vi "Rawdata_Analyzer.vi"() -> ()   [LabVIEW 2020]
uses:
  ctl/Image_RAW_Bayer_Pattern.ctl
  ctl/Image_Configuration.ctl
  <vilib>/vision/Image Controls.llb/IMAQ Image.ctl
  <vilib>/Analysis/NI_AALBase.lvlib
panel:
  in  "stop":bool
  out "Current Color Histogram":cluster{"R":u8, "G":u8, "B":u8}
  out "Current Timestamp":u64
  out "Current Image":T1(plugin-control)
  out "Progress":dbl(slide) scale=0.0..100.0
  out "Frame Color Histogram":cluster{"R":u8, "G":u8, "B":u8}[](array[cluster])
  in  "Image Configuration":T2={"Width"=3840, "Height"=2160}
  in  "Bayer Pattern":T3=enum."RGGB (GRBG)"
  in  "Analyze Color?":bool
  in  "Analyze Timestamp?":bool=TRUE
  out "error out":errorcluster
  out "Frame Timestamp (ns)":u64[](array[numeric])
  out "Bytes per Frame":u32
  out "Total Frame Num":i64
  in  "RAWdata File Path":path
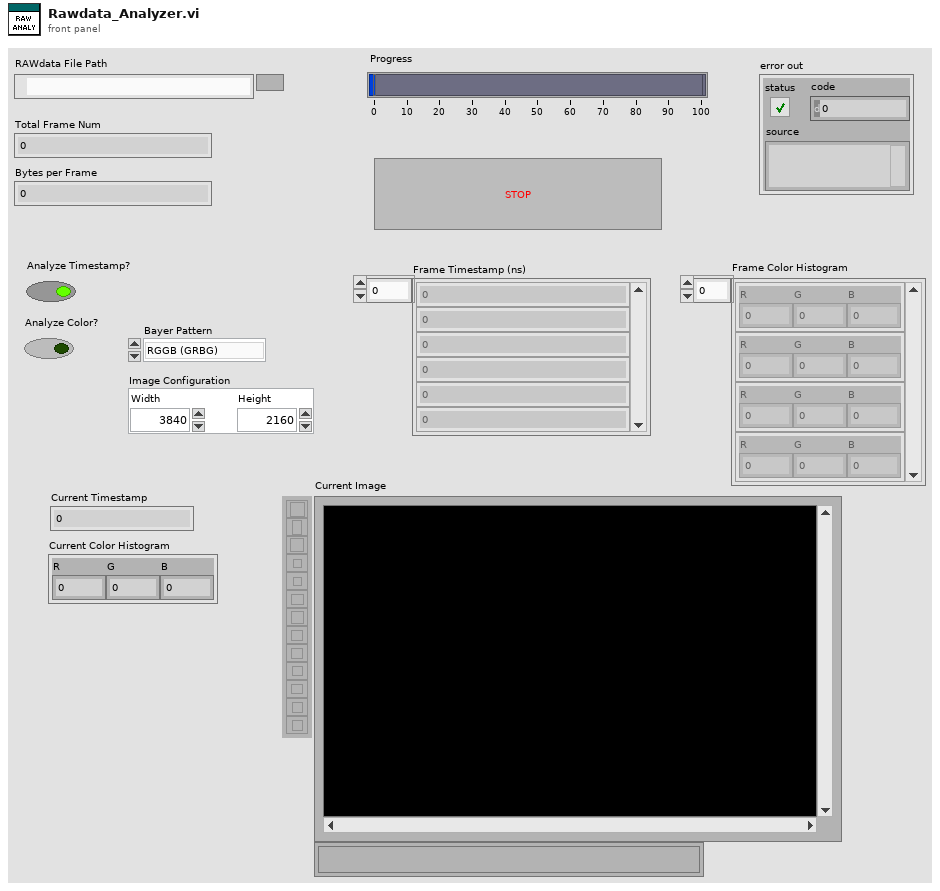
[diagram p1: front panel]
types:
  T1 = typedef "IMAQ Image.ctl" = refnum<image>
  T2 = typedef "Image_Configuration.ctl" = cluster{"Width":i32, "Height":i32}
  T3 = typedef "Image_RAW_Bayer_Pattern.ctl" = enum16{"GBRG (BGGR)", "GRBG (RGGB)", "BGGR (GBRG)", "RGGB (GRBG)", "CRBC (RCCB)"}
  T4 = typedef "Image_Data_Config.ctl" = cluster{"Lines of Image Data":u16, "Bytes per Even Line":u16, "Bytes per Odd Line":u16, "Image Data Type":u8, "Total Image Data Block Size":u32, "Image Data Block Offset":u32}
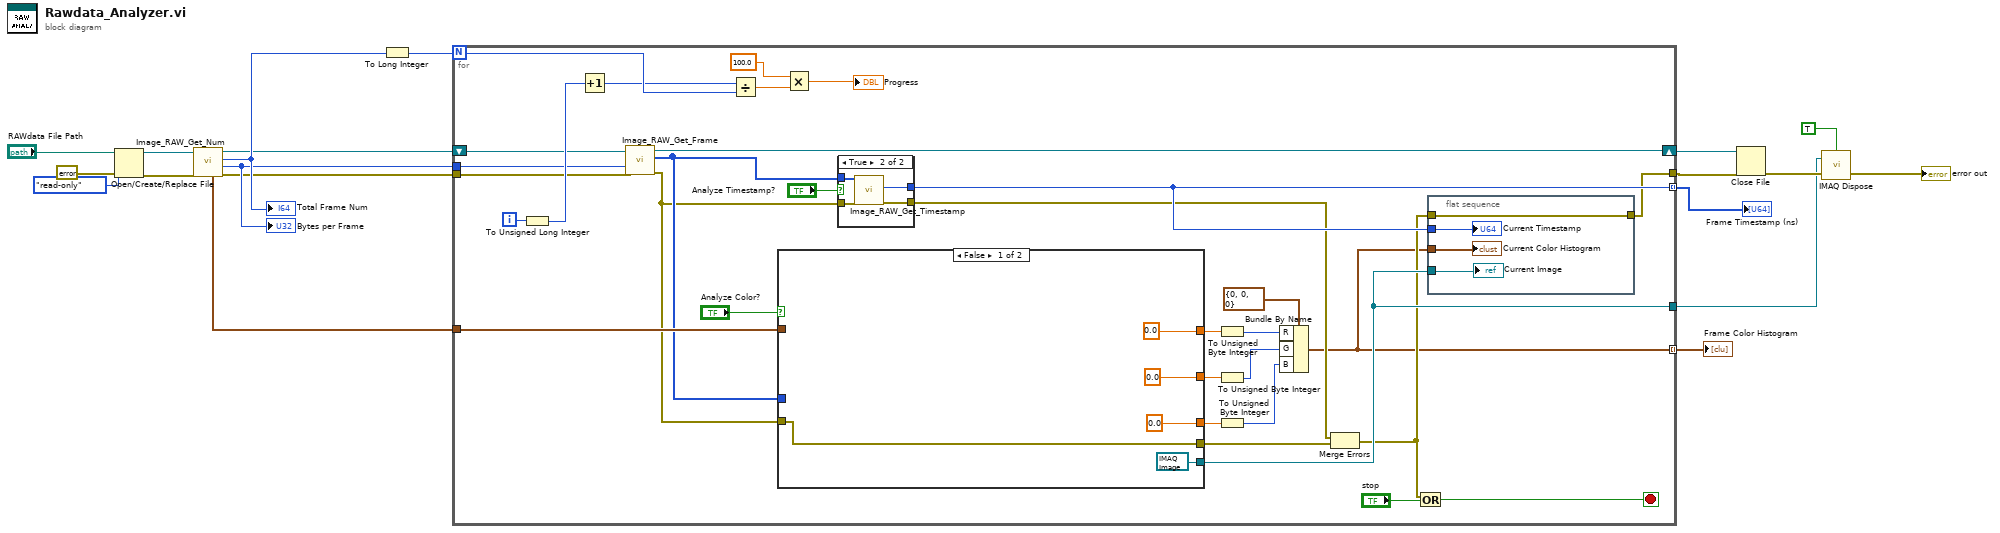
[diagram p0: block diagram]
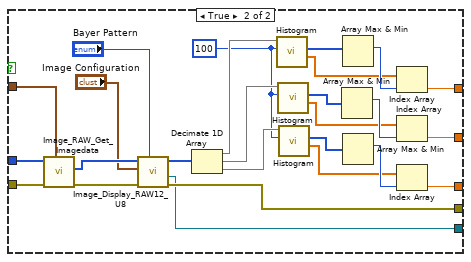
[diagram p2: hidden frame]
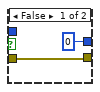
[diagram p3: hidden frame]
diagram:
  n1 = Open/Create/Replace File(file path (use dialog)="RAWdata File Path", error in=errorcluster {"status"=FALSE, "code"=0, "source"=""}, access (0:read/write)=enum16{"read/write", "read-only", "write-only"}."read-only") -> (refnum out=w18:refnum<file>, error out=w17:errorcluster)  [unwired: 3 in, 1 out]
  n2 = call "Image_RAW_Get_Num.vi"("error in (no error)"=w17, "RAW refnum In"=w18) -> ("error out"=w10:errorcluster, "Bytes per Frame"=w11:u32, "Total Frame Num"=w15:i64, "RAW refnum Out"=w12:refnum<file>, "Image Data Config"=w9:T4)  [unwired: 4 in, 1 out]
  "Total Frame Num" <- w15
  "Bytes per Frame" <- w11
  n3 = To Long Integer(number=w15) -> (32bit integer=w14:i32)
  n4 = for {
    N: w14 -> [w46]
    tunnel: w10 -> [w39]
    tunnel: w11 -> [w38]
    tunnel: [w36] -> w8 mode=indexing
    tunnel: w9 -> [w50]
    tunnel: [w41] -> w6
    shift-right: [w37] -> w13
    shift-left: w12 -> [w40]
    tunnel: [w21] -> w3
    tunnel: [w20] -> w2 mode=indexing
    i -> [w51]
    stop <- w44 stop-if-true
    n5 = To Unsigned Long Integer(number=w51) -> (unsigned 32bit integer=w43:u32)
    n6 = Increment(x=w43) -> (x+1=w42:u32)
    n7 = call "Image_RAW_Get_Frame.vi"("error in (no error)"=w39, "Bytes per Frame"=w38, "RAW refnum In"=w40) -> ("error out"=w25:errorcluster, "Frame (U8)"=w26:u8[], "RAW refnum Out"=w37:refnum<file>)  [unwired: 6 in]
    n8 = Divide(x=w42, y=w46) -> (x/y=w48:dbl)
    n9 = case shown="False" "Analyze Color?" {
      tunnel: w50 -> [_ w82]
      tunnel: [0.0 w63] -> w32
      tunnel: [0.0 w62] -> w31
      tunnel: [0.0 w61] -> w30
      tunnel: [w52 w60] -> w24
      tunnel: [T1 refnum ("Image") w59] -> w41
      tunnel: w26 -> [_ w58]
      tunnel: w25 -> [w52 w57]
      frame False {
      }
      frame True {
        w73 = 100 ("intervals")
        n10 = call "Image_RAW_Get_Imagedata.vi"("Image Data Config"=w82, "error in (no error)"=w57, "Frame (U8)"=w58) -> ("error out"=w79:errorcluster, "Image Data Payload"=w81:u8[])  [unwired: 7 in]
        n11 = call "Image_Display_RAW12_U8.vi"("Bayer Pattern"="Bayer Pattern", "error in (no error)"=w79, "Image Configuration"="Image Configuration", "RAW12 Frame (U8)"=w81) -> ("error out"=w60:errorcluster, "Image"=w59:T1, "RGB Frame Out"=w77:u8[])  [unwired: 4 in, 1 out]
        n12 = Decimate 1D Array(w77) -> (w76:u8[], w75:u8[], w74:u8[])
        n13 = call <vilib>:"Histogram.vi"("intervals"=w73, "X"=w76) -> ("X Values"=w66:dbl[], "Histogram: h(x)"=w69:i32[])  [unwired: 6 in, 2 out]
        n14 = call <vilib>:"Histogram.vi"("intervals"=w73, "X"=w75) -> ("X Values"=w65:dbl[], "Histogram: h(x)"=w68:i32[])  [unwired: 6 in, 2 out]
        n15 = call <vilib>:"Histogram.vi"("intervals"=w73, "X"=w74) -> ("X Values"=w64:dbl[], "Histogram: h(x)"=w67:i32[])  [unwired: 6 in, 2 out]
        n16 = Array Max & Min(array=w68) -> (max index (indices)=w71:i32)  [unwired: 3 out]
        n17 = Array Max & Min(array=w69) -> (max index (indices)=w72:i32)  [unwired: 3 out]
        n18 = Array Max & Min(array=w67) -> (max index (indices)=w70:i32)  [unwired: 3 out]
        n19 = Index Array(array=w66, index=w72) -> (element=w63:dbl)
        n20 = Index Array(array=w65, index=w71) -> (element=w62:dbl)
        n21 = Index Array(array=w64, index=w70) -> (element=w61:dbl)
      }
    }
    n22 = Multiply(x=100.0, y=w48) -> (x*y=→"Progress":dbl)
    n23 = case shown="True" "Analyze Timestamp?" {
      tunnel: [u64 0 ("Frame Timestamp") w88] -> w36
      tunnel: w26 -> [_ w87]
      tunnel: w25 -> [w84 w86]
      tunnel: [w84 w85] -> w23
      frame False {
      }
      frame True {
        n24 = call "Image_RAW_Get_Timestamp.vi"("error in (no error)"=w86, "Frame (U8)"=w87) -> ("error out"=w85:errorcluster, "Frame Timestamp"=w88:u64)  [unwired: 8 in]
      }
    }
    n25 = To Unsigned Byte Integer(number=w32) -> (unsigned 8bit integer=w29:u8)
    n26 = To Unsigned Byte Integer(number=w31) -> (unsigned 8bit integer=w28:u8)
    n27 = To Unsigned Byte Integer(number=w30) -> (unsigned 8bit integer=w27:u8)
    n28 = Bundle By Name(cluster=cluster{"R":u8, "G":u8, "B":u8} {"R"=0, "G"=0, "B"=0} ("Frame Color Histogram"), "R"=w29, "G"=w28, "B"=w27) -> (w20:cluster{"R":u8, "G":u8, "B":u8})
    n29 = Merge Errors(w23, w24) -> (w22:errorcluster)
    n30 = Or(x=w22, y="stop") -> (x .or. y?=w44:bool)
    n31 = flat-sequence {
      tunnel: w22 -> [w92]
      tunnel: [w92] -> w21
      tunnel: w36 -> [w91]
      tunnel: w20 -> [w89]
      tunnel: w41 -> [w90]
      frame #0 {
        "Current Timestamp" <- w91
        "Current Color Histogram" <- w89
        "Current Image" <- w90
      }
    }
  }
  "Frame Timestamp (ns)" <- w8
  "Frame Color Histogram" <- w2
  n32 = Close File(refnum=w13, error in=w3) -> (error out=w7:errorcluster)  [unwired: 1 out]
  n33 = call "IMAQ Dispose"("All Images? (No)"=TRUE, "Image"=w6, "error in (no error)"=w7) -> ("error out"=→"error out":errorcluster)  [unwired: 3 in]
